vi "WriteExternalInterfaces.vi"(8 "ErrorIn":errorcluster, 10 "ExternalInterfaces":T1[](array[typedef]), 11 "YAFFooterIn":refnum<class "YAFFooter.lvclass">) -> (0 "ErrorOut":errorcluster, 3 "YAFFooterOut":refnum<class "YAFFooter.lvclass">)   [LabVIEW 2021, in "YAFFooter.lvlib" / "YAFFooter.lvclass"]
uses:
  YAFFooter.lvclass
  Library_TAF_Support/ClusterArrayConversion/BundledArray.ctl
  YAFFooter.lvclass/YAFFooter.ctl
  0f9fbe56-9f9a-4601-8b43-1fc07a995cee.vi
  0f9fbe56-9f9a-4601-8b43-1fc07a995cee.vi/e733eca7-9823-4359-8665-3b184f9a7377.vi
  0f9fbe56-9f9a-4601-8b43-1fc07a995cee.vi/185eb5ab-e8f7-4395-854b-f566a9b9020c.vi
  <vilib>/Utility/Data Type/Get Cluster Information.vi
  <vilib>/Utility/Data Type/Get Type Information.vi
  <userlib>/_OpenG.lib/lvdata/lvdata.llb/Array of VData to VCluster__ogtk.vi
  <vilib>/Utility/LVClass/Get LV Class Name.vi
  Interface_TAF_TraceSubscriptor/ITAFFilteredTrace/ITAFFilteredTrace.lvclass
  Library_TAF_Support/ClusterArrayConversion/ClusterArrayConversion.lvlib
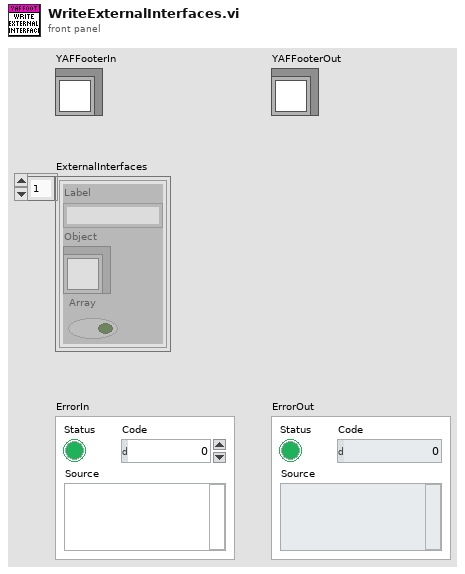
[diagram p1: front panel]
types:
  T1 = typedef "ClusterArrayConversion.lvlib/BundledArray.ctl" = cluster{"Label":string, "Object":refnum<class>, "Array":bool}
  T2 = cluster{"TracerSource":refnum<class "ITAFFilteredTrace.lvclass">}
  T3 = typedef "TAFTraceWindow.lvclass/FilterConfiguration.ctl" = cluster{"TraceColumn":i32, "FilterFunction":T4, "SearchText":string}
  T4 = typedef "TAFTraceWindow.lvclass/FilterFunction.ctl" = enum16{"Exact", "Regex"}
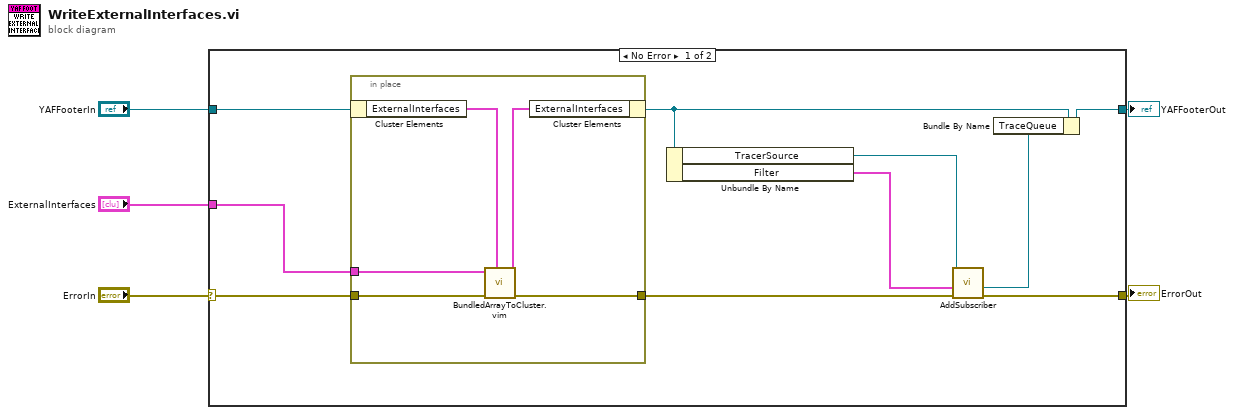
[diagram p0: block diagram]
diagram:
  n1 = case shown="No Error" "ErrorIn" {
    selector: "ErrorIn" -> [w15 w22]
    tunnel: [w13 w22] -> w4
    tunnel: [w8 w21] -> w2
    tunnel: "YAFFooterIn" -> [w12 w21]
    tunnel: "ExternalInterfaces" -> [w11 _]
    frame No Error {
      n2 = in-place {
        in-place-border: [w20] -> w14
        in-place-border: w15 -> [w19]
        in-place-border: w11 -> [w18]
        n3 = in-place-cluster #1(w12) -> ("ExternalInterfaces"=w17:T2)
        n4 = call "BundledArrayToCluster.vim"("Type"=w17, "ErrorIn"=w19, "BundeledLabels"=w18) -> ("ErrorOut"=w20:errorcluster, "DataOut"=w16:T2)  [unwired: 7 in]
        n5 = in-place-cluster #1("ExternalInterfaces"=w16) -> (w10:refnum<class "YAFFooter.lvclass">)
      }
      n6 = Unbundle By Name(w10) -> ("TracerSource"=w9:refnum<class "ITAFFilteredTrace.lvclass">, "Filter"=w6:T3[])
      n7 = call-dynamic "AddSubscriber.vi"("ErrorIn"=w14, "Filters"=w6, "ITAFFilteredTrace in"=w9) -> ("ErrorOut"=w13:errorcluster, "TraceQueue"=w7:refnum<queue>)  [unwired: 6 in, 1 out]
      n8 = Bundle By Name(cluster=w10, "TraceQueue"=w7) -> (w8:refnum<class "YAFFooter.lvclass">)
    }
    frame Error {
    }
  }
  "ErrorOut" <- w4
  "YAFFooterOut" <- w2
